vi "Connect Standalone Wlan Card.vi"(8 "error in (no error)":errorcluster, 10 "path in":path=path "D:/Cobham_QCA9984/DUT/dut_control/QCA_DUT_Func.dll", 11 "DUT_IP":string) -> (0 "error out":errorcluster, 2 "return type":u8, 3 "DUT_IP out":string)   [LabVIEW 2015, in "QCA_DUT_Func.lvlib"]
doc: "DLL_QMSL_AEROFLEX bool _stdcall ConnectStandaloneWlanCard(char DUT_IP[30]);"
uses:
  QCA_DUT_Func.lvlib
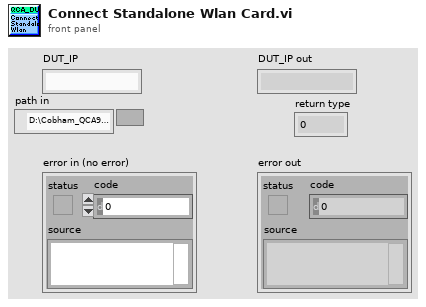
[diagram p1: front panel]
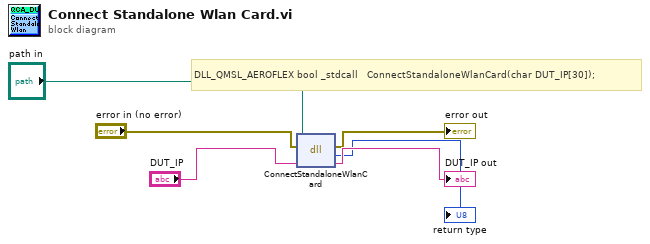
[diagram p0: block diagram]
diagram:
  # "DLL_QMSL_AEROFLEX bool _stdcall   ConnectStandaloneWlanCard(char DUT_IP[30]);"
  n1 = dll-call lib="D:/4-Up-WLAN-Test-System/DUT Control/DUT/dut_control/QCA_DUT_Func.dll" fn="ConnectStandaloneWlanCard"(path in="path in", error in="error in (no error)", "IP"="DUT_IP") -> (error out=→"error out":errorcluster, "return type"=→"return type":i32, "IP"=→"DUT_IP out":string)  [unwired: 1 in, 1 out]
